vi "calculate uptime.vi"() -> ()   [LabVIEW 2018]
uses:
  <vilib>/Utility/file.llb/Read Delimited Spreadsheet (string).vi
panel:
  out "files":path[](array[path])
  out "Array":string[][](array[string])
  out "% up time":dbl format="%.2f%%"
  out "total running time":dbl format="%<%W weeks, %D days, %H hours, %M minutes>t"
  out "total up time":dbl format="%<%W weeks, %D days, %H hours, %M minutes>t"
  out "Waveform Graph":dbl[](graph)
  out "total running time bad":timestamp
  in  "Card.Channel":dbl=8.04
  in  "End":cluster{"Run":i32, "Subrun":i32}={"Run"=310, "Subrun"=-1}
  in  "Start":cluster{"Run":i32, "Subrun":i32}={"Run"=280, "Subrun"=0}
  out "Timestamp Array":timestamp[](array[timestamp])
  out "Plot":cluster{timestamp[], dbl[]}(graph)
  # "channel must have 2 significant figures!"
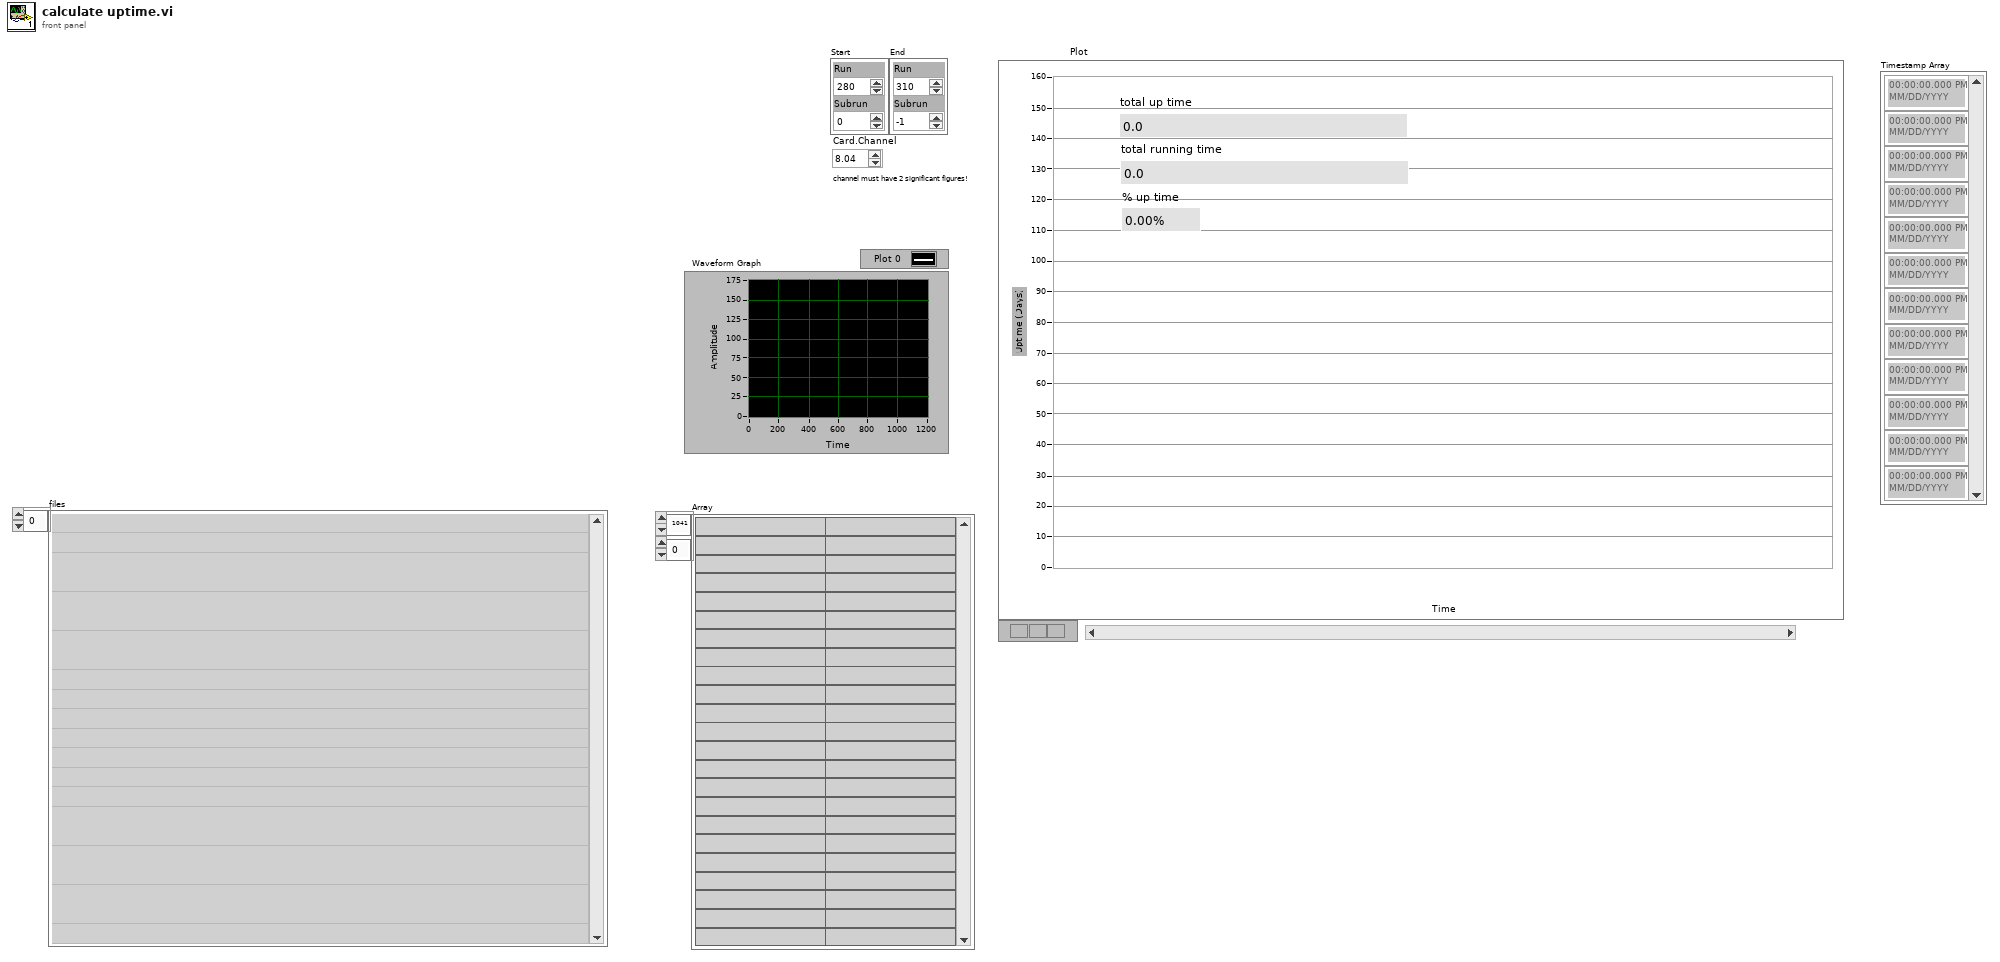
[diagram p1: front panel]
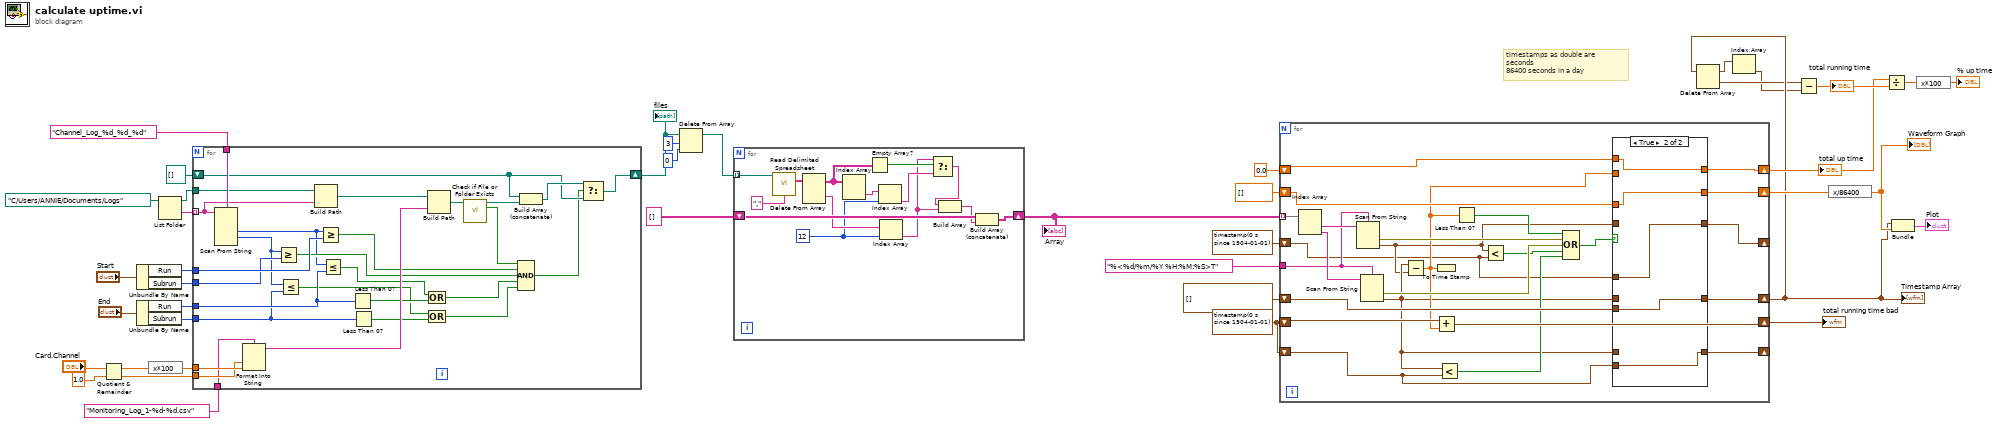
[diagram p0: block diagram]
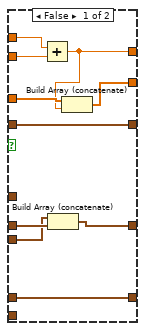
[diagram p2: hidden frame]
diagram:
  w9 = timestamp(0 s since 1904-01-01)
  # "timestamps as double are seconds\n86400 seconds in a day"
  n1 = Quotient & Remainder(x="Card.Channel", y=1.0) -> (x-y*floor(x/y)=w25:dbl, floor(x/y)=w28:dbl)
  n2 = Unbundle By Name("Start") -> ("Run"=w35:i32, "Subrun"=w34:i32)
  n3 = Unbundle By Name("End") -> ("Run"=w33:i32, "Subrun"=w32:i32)
  n4 = expression code="x*100"(w25) -> (w24:dbl)
  n5 = List Folder(path=path "C:/Users/ANNIE/Documents/Logs" ("file path (dialog if empty)")) -> (path out=w30:path, folder names=w40:string[])  [unwired: 3 in, 2 out]
  n6 = for {
    tunnel: w40 -> [w66] mode=indexing
    tunnel: w35 -> [w69]
    tunnel: w34 -> [w68]
    tunnel: w33 -> [w57]
    tunnel: w32 -> [w56]
    tunnel: "Channel_Log_%d_%d_%d" ("format string") -> [w70]
    shift-right: [w64] -> w6
    shift-left: path[] [] -> [w58]
    tunnel: w30 -> [w67]
    tunnel: w24 -> [w63]
    tunnel: w28 -> [w62]
    tunnel: "Monitoring_Log_1-%d-%d.csv" ("format string") -> [w61]
    n7 = Scan From String(format string=w70, input string=w66) -> (output 1=w44:i32, output 2=w45:i32)  [unwired: 6 in, 3 out]
    n8 = Format Into String(format string=w61, w62, w63) -> (resulting string=w60:string)  [unwired: 2 in, 1 out]
    n9 = Greater Or Equal?(x=w45, y=w68) -> (x >= y?=w48:bool)
    n10 = Less Or Equal?(x=w45, y=w56) -> (x <= y?=w53:bool)
    n11 = Build Path(base path=w67, name or relative path=w66) -> (appended path=w59:path)
    n12 = Greater Or Equal?(x=w44, y=w69) -> (x >= y?=w49:bool)
    n13 = Less Or Equal?(x=w44, y=w57) -> (x <= y?=w55:bool)
    n14 = Less Than 0?(x=w57) -> (x < 0?=w54:bool)
    n15 = Less Than 0?(x=w56) -> (x < 0?=w52:bool)
    n16 = Build Path(base path=w59, name or relative path=w60) -> (appended path=w42:path)
    n17 = Compound Arithmetic op=OR(w55, w54) -> (w47:bool)
    n18 = Compound Arithmetic op=OR(w53, w52) -> (w46:bool)
    n19 = call <vilib>:"Check if File or Folder Exists.vi"("path"=w42) -> ("file or folder exists?"=w50:bool, "dup path"=w51:path)  [unwired: 8 in, 1 out]
    n20 = Compound Arithmetic op=AND(w50, w49, w48, w47, w46) -> (w43:bool)
    n21 = Build Array (concatenate)(w58, w51) -> (w65:path[])
    n22 = Select(t=w65, s=w43, f=w58) -> (s? t:f=w64:path[])
  }
  "files" <- w6
  n23 = Delete From Array(array=w6, length=3, index=0 ("length")) -> (array with subset deleted=w5:path[])  [unwired: 1 out]
  n24 = for {
    tunnel: w5 -> [w83] mode=indexing
    shift-right: [w82] -> w20
    shift-left: string[][] [] -> [w81]
    w71 = 12 ("index")
    n25 = call-poly <vilib>:"Read Delimited Spreadsheet.vi"("file path (dialog if empty)"=w83, "delimiter (\\t)"="," ("delimiter (\\t)")) -> ("all rows"=w80:string[][])  [unwired: 8 in, 5 out]
    n26 = Delete From Array(array=w80) -> (deleted portion=w77:string[], array with subset deleted=w76:string[][])  [unwired: 3 in]
    n27 = Index Array(array=w76) -> (element=w79:string[])  [unwired: 2 in]
    n28 = Empty Array?(array=w76) -> (empty?=w78:bool)
    n29 = Index Array(array=w79, index=w71) -> (element=w75:string)
    n30 = Index Array(array=w77, index=w71) -> (element=w74:string)
    n31 = Select(t=w74, s=w78, f=w75) -> (s? t:f=w73:string)
    n32 = Build Array(w73, w74) -> (w72:string[])
    n33 = Build Array (concatenate)(w81, w72) -> (w82:string[][])
  }
  "Array" <- w20
  n34 = for {
    tunnel: "%<%d/%m/%Y %H:%M:%S>T" ("format string") -> [w106]
    tunnel: w20 -> [w109] mode=indexing
    shift-right: [w105] -> w21
    shift-left: w9 -> [w104]
    shift-right: [w93] -> w17
    shift-left: 0.0 -> [w95]
    shift-right: [w103] -> w4
    shift-left: timestamp[] [] -> [w102]
    shift-right: [w101] -> w14
    shift-left: dbl[] [] -> [w100]
    shift-right: [w87] -> _
    shift-left: timestamp(0 s since 1904-01-01) -> [w85]
    shift-right: [w89] -> _
    shift-left: w9 -> [w86]
    n35 = Index Array(array=w109) -> (element #1=w107:string, element #2=w108:string)  [unwired: 2 in]
    n36 = Scan From String(format string=w106, input string=w107) -> (error out=w98:errorcluster, output 1=w88:timestamp)  [unwired: 3 in, 2 out]
    n37 = Scan From String(format string=w106, input string=w108) -> (error out=w97:errorcluster, output 1=w90:timestamp)  [unwired: 3 in, 2 out]
    n38 = Subtract(x=w90, y=w88) -> (x-y=w94:dbl)
    n39 = To Time Stamp(1:w94) -> ()  [unwired: 1 out]
    n40 = Add(x=w104, y=w94) -> (x+y=w105:timestamp)
    n41 = Less?(x=w90, y=w86) -> (x < y?=w91:bool)
    n42 = Less Than 0?(x=w94) -> (x < 0?=w99:bool)
    n43 = Less?(x=w88, y=w85) -> (x < y?=w92:bool)
    n44 = Compound Arithmetic op=OR(w99, w98, w97, w92, w91) -> (w96:bool)
    n45 = case shown="True" w96 {
      tunnel: w90 -> [w119 _]
      tunnel: [w118 w122] -> w103
      tunnel: w102 -> [w117 w122]
      tunnel: [w116 w123] -> w101
      tunnel: w100 -> [w115 w123]
      tunnel: w95 -> [w114 w124]
      tunnel: w94 -> [w113 _]
      tunnel: [w112 w124] -> w93
      tunnel: [w111 w121] -> w89
      tunnel: w90 -> [w111 _]
      tunnel: w88 -> [w110 _]
      tunnel: [w110 w120] -> w87
      tunnel: w86 -> [_ w121]
      tunnel: w85 -> [_ w120]
      frame False {
        n46 = Add(x=w114, y=w113) -> (x+y=w112:dbl)
        n47 = Build Array (concatenate)(w117, w119) -> (w118:timestamp[])
        n48 = Build Array (concatenate)(w115, w112) -> (w116:dbl[])
      }
      frame True {
      }
    }
  }
  "Timestamp Array" <- w4
  "total running time bad" <- w21
  "total up time" <- w17
  n49 = Delete From Array(array=w4) -> (deleted portion=w3:timestamp, array with subset deleted=w2:timestamp[])  [unwired: 2 in]
  n50 = Index Array(array=w2) -> (element=w1:timestamp)  [unwired: 1 in]
  n51 = Subtract(x=w3, y=w1) -> (x-y=w18:dbl)
  "total running time" <- w18
  n52 = expression code="x/86400"(w14) -> (w13:dbl[])
  "Waveform Graph" <- w13
  n53 = Divide(x=w17, y=w18) -> (x/y=w16:dbl)
  n54 = Bundle(w4, w13) -> (→"Plot":cluster{timestamp[], dbl[]})  [unwired: 1 in]
  n55 = expression code="x*100"(w16) -> (→"% up time":dbl)
